vi "Copy .LLB to NI VeriStand dir.vi"(5 "Files Generated by Build":path[](array[path]), 6 "Top Level/Always Included VIs":path[](array[path]), 7 "Destination Path":path, 8 "error in (no error)":errorcluster, 9 "Target Name":string, 10 "Build Specification Name":string, 11 "Project Path":path) -> (0 "error out":errorcluster)   [LabVIEW 2017]
doc: "This VI is called after each run of a build specification. The VI will copy the generated LLB (Engine or System Explorer) into the VeriStand Custom Device folder (...\\Documents\\National Instruments\\NI VeriStand 2013...)."
uses:
  <vilib>/Utility/sysdir.llb/System Directory Type.ctl
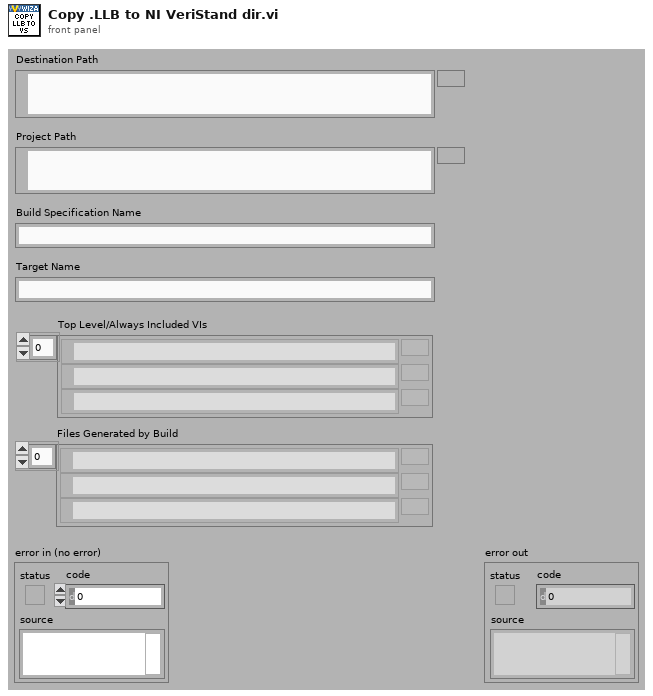
[diagram p1: front panel]
types:
  T1 = typedef "System Directory Type.ctl" = i32
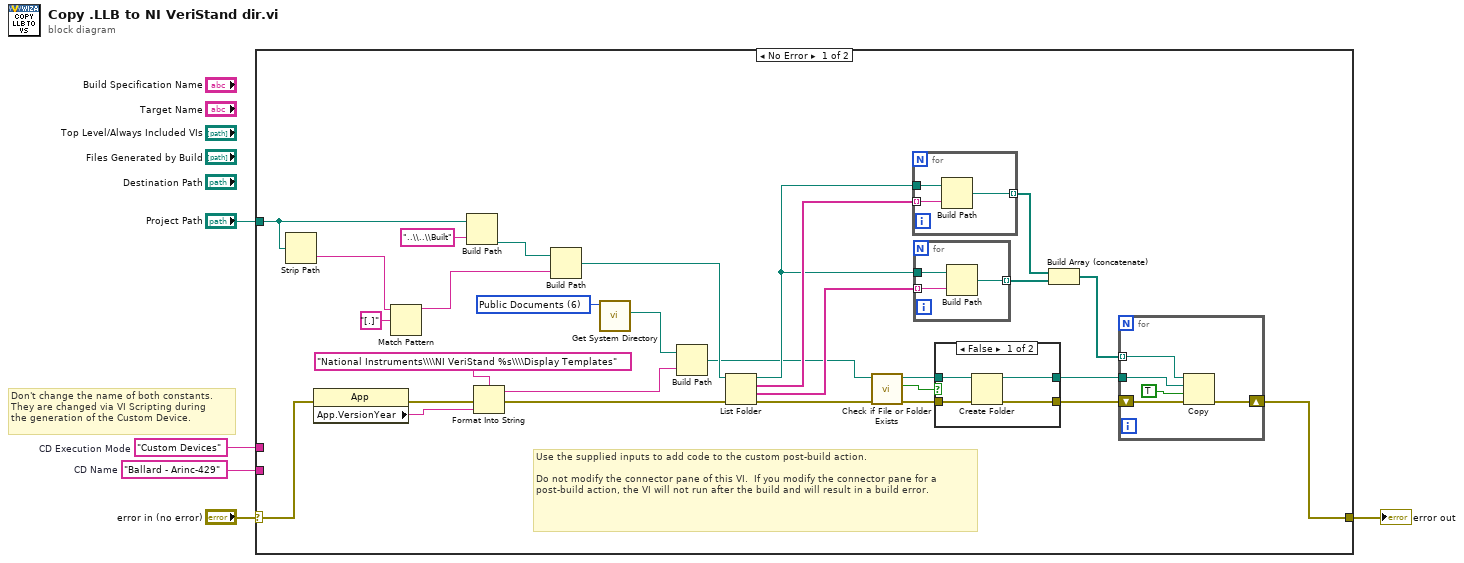
[diagram p0: block diagram]
diagram:
  w2 = "Ballard - Arinc-429"  # CD Name
  w3 = "Custom Devices"  # CD Execution Mode
  # "Don't change the name of both constants.\nThey are changed via VI Scripting during\nthe generation of the Custom Device."
  n1 = case shown="No Error" "error in (no error)" {
    selector: "error in (no error)" -> [w14 w52]
    tunnel: [w16 w52] -> w1
    tunnel: "Project Path" -> [w9 _]
    tunnel: w3 -> [_ _]
    tunnel: w2 -> [_ _]
    frame No Error {
      w20 = T1 6 items=["User Home"=0, "User Desktop"=1, "User Documents"=2, "User Application Data"=3, "User Preferences"=4, "User Temporary"=5, "Public Documents"=6, "Public Application Data"=7, "Public Preferences"=8, "Public Cache"=13, "System Core Libraries"=9, "System Installed Libraries"=10, "Application Files"=11, "Boot Volume Root"=12] ("system directory type")
      # "Use the supplied inputs to add code to the custom post-build action.\n\nDo not modify the connector pane of this VI.  If you modify the connector pane for a post-build action, the VI will not run after the build and will result in a build error."
      n2 = Strip Path(path=w9) -> (name=w8:string)  [unwired: 1 out]
      n3 = property class="App"(error in=w14) -> (error out=w19:errorcluster, "App.VersionYear"=w18:string)  [unwired: 1 in, 1 out]
      n4 = Match Pattern(string=w8, regular expression="[.]") -> (before substring=w7:string)  [unwired: 1 in, 3 out]
      n5 = Build Path(base path=w9, name or relative path="..\\..\\Built") -> (appended path=w23:path)
      n6 = Format Into String(format string="National Instruments\\\\NI VeriStand %s\\\\Display Templates" ("name or relative path"), error in=w19, w18) -> (resulting string=w22:string, error out=w13:errorcluster)  [unwired: 1 in]
      n7 = Build Path(base path=w23, name or relative path=w7) -> (appended path=w25:path)
      n8 = call <vilib>:"Get System Directory.vi"("system directory type"=w20) -> ("system directory"=w21:path)  [unwired: 10 in]
      n9 = Build Path(base path=w21, name or relative path=w22) -> (appended path=w15:path)
      n10 = List Folder(path=w25, error in=w13) -> (path out=w27:path, filenames=w34:string[], folder names=w28:string[], error out=w24:errorcluster)  [unwired: 2 in]
      n11 = call <vilib>:"Check if File or Folder Exists.vi"("error in (no error)"=w24, "path"=w15) -> ("error out"=w29:errorcluster, "file or folder exists?"=w31:bool, "dup path"=w30:path)  [unwired: 7 in]
      n12 = for {
        tunnel: w34 -> [w50] mode=indexing
        tunnel: w27 -> [w51]
        tunnel: [w49] -> w33 mode=indexing
        n13 = Build Path(base path=w51, name or relative path=w50) -> (appended path=w49:path)
      }
      n14 = for {
        tunnel: w28 -> [w47] mode=indexing
        tunnel: w27 -> [w48]
        tunnel: [w46] -> w26 mode=indexing
        n15 = Build Path(base path=w48, name or relative path=w47) -> (appended path=w46:path)
      }
      n16 = case shown="False" w31 {
        tunnel: w30 -> [w38 w40]
        tunnel: w29 -> [w37 w39]
        tunnel: [w36 w40] -> w11
        tunnel: [w35 w39] -> w10
        frame False {
          n17 = Create Folder(path (use dialog)=w38, error in=w37) -> (created path=w36:path, error out=w35:errorcluster)  [unwired: 1 in, 1 out]
        }
        frame True {
        }
      }
      n18 = Build Array (concatenate)(w33, w26) -> (w32:path[])
      n19 = for {
        tunnel: w32 -> [w42] mode=indexing
        shift-right: [w43] -> w16
        shift-left: w10 -> [w44]
        tunnel: w11 -> [w41]
        n20 = Copy(8:w44, 9:TRUE ("overwrite (F)"), 10:w41, 11:w42) -> (0:w43:errorcluster)  [unwired: 1 in, 2 out]
      }
    }
    frame Error {
    }
  }
  "error out" <- w1
